vi "Get URI String.vi"(8 "error in (no error)":errorcluster, 11 "URI in":refnum<class "URI.lvclass">) -> (0 "error out":errorcluster, 2 "URI String":string, 3 "URI out":refnum<class "URI.lvclass">)   [LabVIEW 2020, in "URI.lvclass"]
uses:
  URI.lvclass
  URI.lvclass/URI.ctl
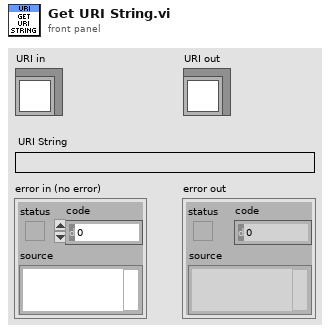
[diagram p1: front panel]
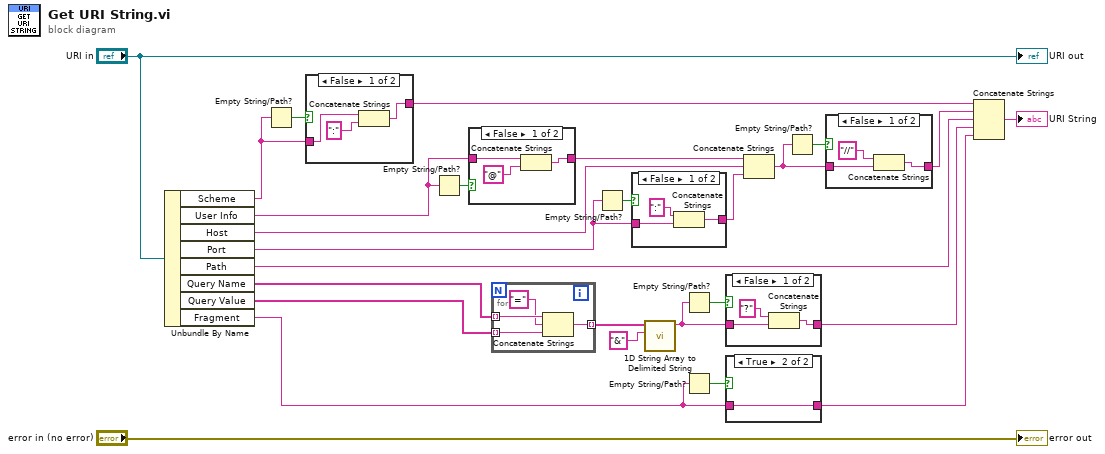
[diagram p0: block diagram]
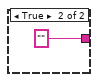
[diagram p6: hidden frame]
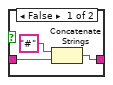
[diagram p7: hidden frame]
diagram:
  n1 = Unbundle By Name("URI in") -> ("Scheme"=w25:string, "User Info"=w2:string, "Host"=w21:string, "Port"=w23:string, "Path"=w16:string, "Query Name"=w15:string[], "Query Value"=w14:string[], "Fragment"=w7:string)
  n2 = Empty String/Path?(string/path=w25) -> (empty?=w26:bool)
  n3 = case shown="False" w26 {
    tunnel: w25 -> [w30 _]
    tunnel: [w28 ""] -> w18
    frame False {
      n4 = Concatenate Strings(w30, ":" ("string")) -> (w28:string)
    }
    frame True {
    }
  }
  n5 = Empty String/Path?(string/path=w2) -> (empty?=w3:bool)
  n6 = case shown="False" w3 {
    tunnel: w2 -> [w34 w35]
    tunnel: [w32 w35] -> w4
    frame False {
      n7 = Concatenate Strings(w34, "@" ("string")) -> (w32:string)
    }
    frame True {
    }
  }
  n8 = for {
    tunnel: w15 -> [w39] mode=indexing
    tunnel: w14 -> [w38] mode=indexing
    tunnel: [w36] -> w13 mode=indexing
    n9 = Concatenate Strings(w39, "=" ("string"), w38) -> (w36:string)
  }
  n10 = Empty String/Path?(string/path=w23) -> (empty?=w24:bool)
  n11 = case shown="False" w24 {
    tunnel: w23 -> [w42 w43]
    tunnel: [w40 w43] -> w22
    frame False {
      n12 = Concatenate Strings(":" ("string"), w42) -> (w40:string)
    }
    frame True {
    }
  }
  n13 = call <vilib>:"1D String Array to Delimited String.vi"("delimiter"="&", "string array"=w13) -> ("delimited string"=w10:string)  [unwired: 9 in]
  n14 = Empty String/Path?(string/path=w10) -> (empty?=w11:bool)
  n15 = Empty String/Path?(string/path=w7) -> (empty?=w8:bool)
  n16 = case shown="False" w11 {
    tunnel: w10 -> [w46 w47]
    tunnel: [w44 w47] -> w9
    frame False {
      n17 = Concatenate Strings("?" ("string"), w46) -> (w44:string)
    }
    frame True {
    }
  }
  n18 = case shown="True" w8 {
    tunnel: w7 -> [w50 w51]
    tunnel: [w48 w51] -> w6
    frame False {
      n19 = Concatenate Strings("#" ("string"), w50) -> (w48:string)
    }
    frame True {
    }
  }
  n20 = Concatenate Strings(w4, w21, w22) -> (w19:string)
  n21 = Empty String/Path?(string/path=w19) -> (empty?=w20:bool)
  n22 = case shown="False" w20 {
    tunnel: w19 -> [w54 w55]
    tunnel: [w52 w55] -> w17
    frame False {
      n23 = Concatenate Strings("//" ("string"), w54) -> (w52:string)
    }
    frame True {
    }
  }
  n24 = Concatenate Strings(w18, w17, w16, w9, w6) -> (→"URI String":string)
  "error out" <- "error in (no error)"
  "URI out" <- "URI in"
